vi "Timer Core.vi"(0 "timer":T2, 1 "function":T3(ring)=enum."test ref", 5 "return exisiting (F)":bool, 7 "Accuracy":enum16{"1 ms", "10 ms"}(ring), 9 "name":string, 11 "error in (no error)":errorcluster, 12 "Wait timeout [sec]":dbl format="%.3f") -> (2 "error":i32, 4 "timer out":T2, 6 "Keep Waiting":bool, 8 "Timers out":T1(array[cluster]) {"Total time [sec]" format="%.3f"; "Start time [sec]" format="%.3f"}, 10 "name out":string, 14 "message out":string, 15 "error out":errorcluster)   [LabVIEW 2011]
uses:
  Timer Refnum.ctl
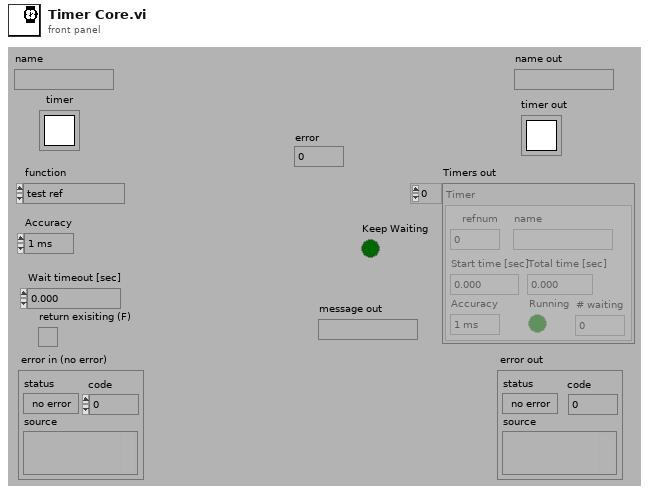
[diagram p1: front panel]
types:
  T1 = cluster{"refnum":u32, "Start time [sec]":dbl, "Running":bool, "Total time [sec]":dbl, "name":string, "Accuracy":enum16{"1 ms", "10 ms"}, "# waiting":i32}[]
  T2 = typedef "Timer Refnum.ctl" = refnum<k1>
  T3 = enum16{"open ref", "lookup ref", "close ref", "test ref", "start", "stop", "wait", "reset", "increment # waiting", "decrement #waiting"}
  T4 = enum16{"open ref", "lookup ref", "close ref", "test ref", "start", "stop", "wait", "reset"}
  T5 = cluster{"refnum":u32, "Start time (s)":dbl, "Running":bool, "Total time (s)":dbl, "name":string, "Accuracy":enum16{"1 ms", "10 ms"}, "# waiting":i32}
  T6 = cluster{"refnum":u32, "Start time (s)":dbl, "Running":bool, "Total time (s)":dbl, "name":string, "Accuracy":enum16{"1 ms", "10 ms"}, "# waiting":i32}[]
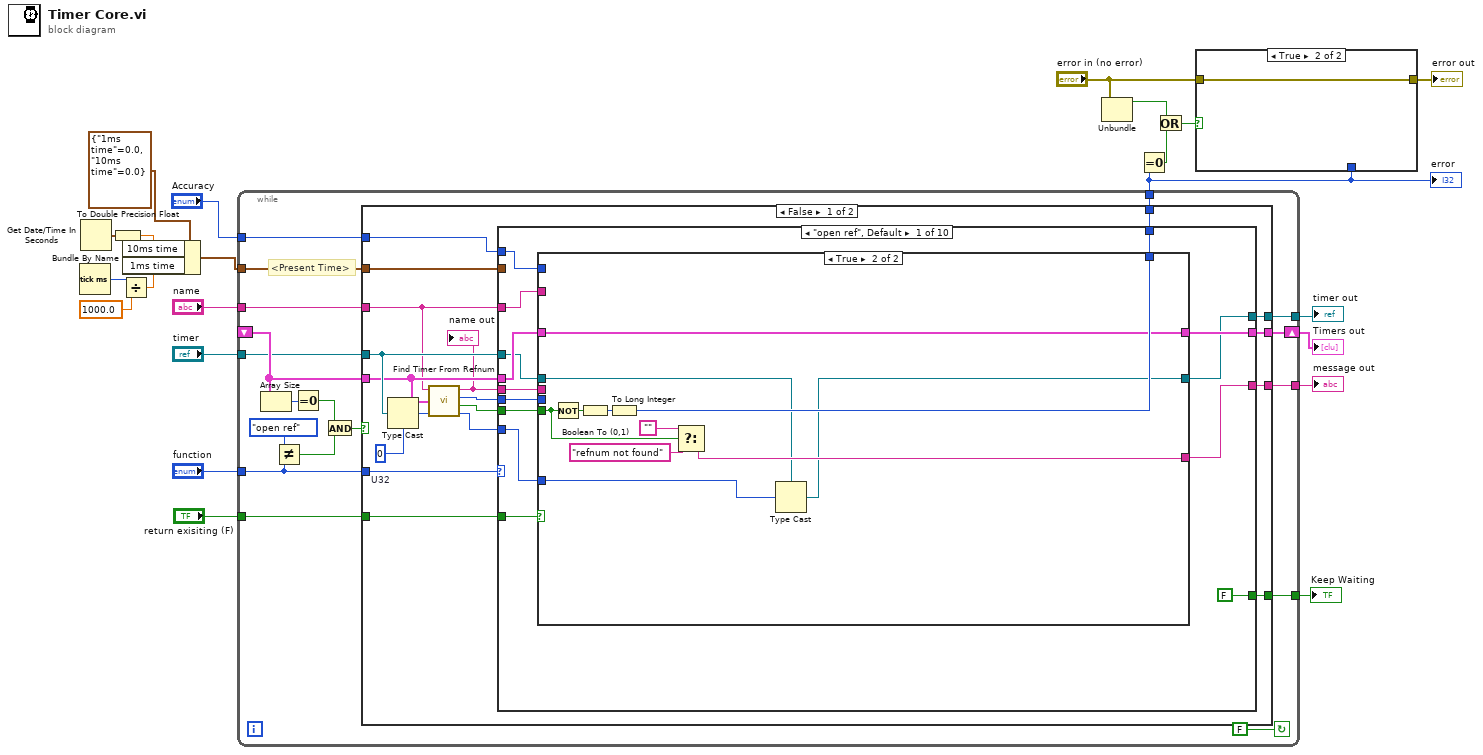
[diagram p0: block diagram]
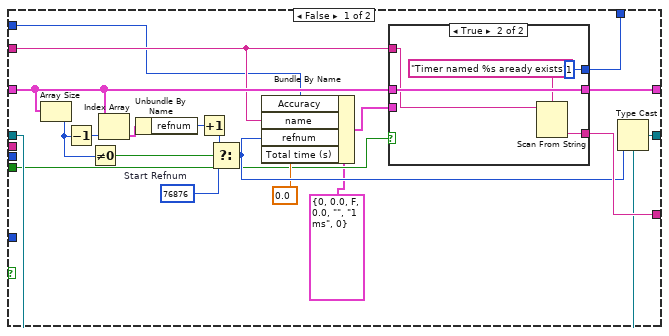
[diagram p2: hidden frame]
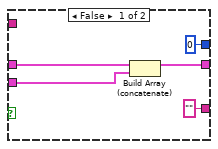
[diagram p3: hidden frame]
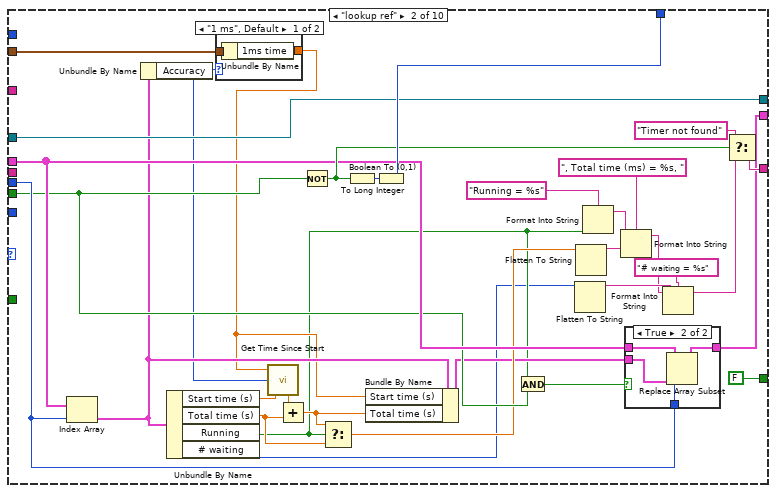
[diagram p4: hidden frame]
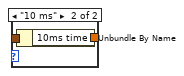
[diagram p5: hidden frame]
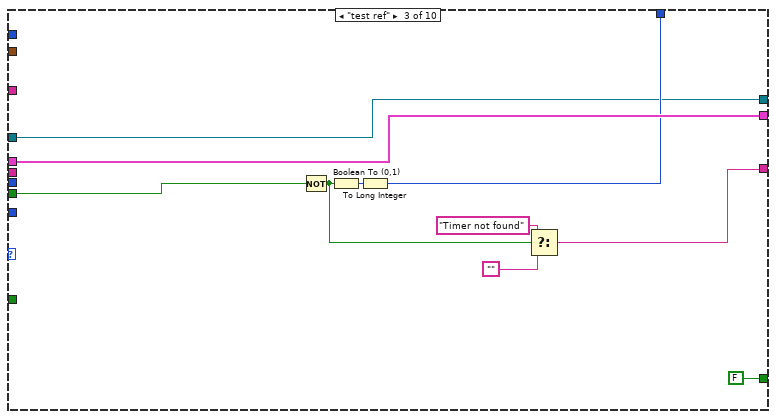
[diagram p7: hidden frame]
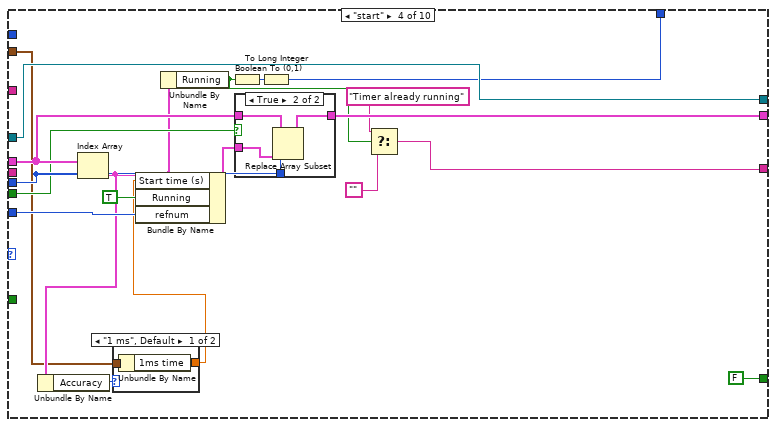
[diagram p8: hidden frame]
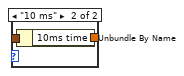
[diagram p9: hidden frame]
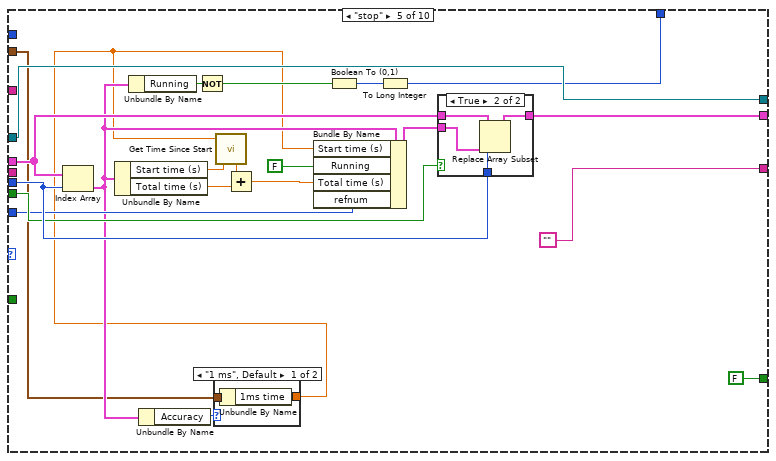
[diagram p11: hidden frame]
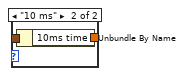
[diagram p12: hidden frame]
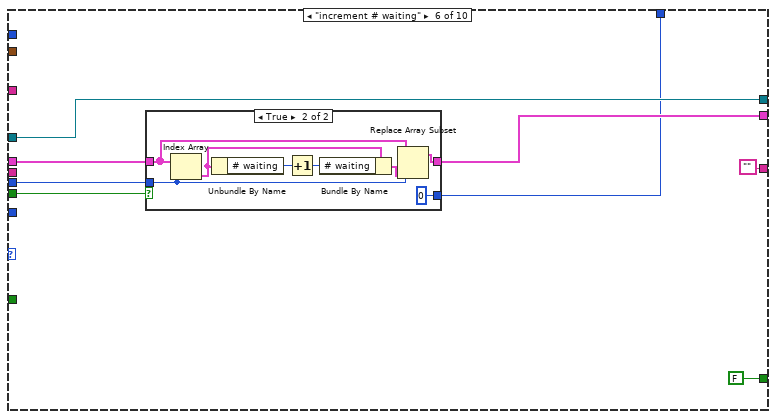
[diagram p14: hidden frame]
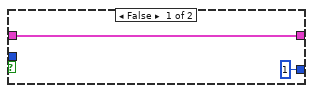
[diagram p15: hidden frame]
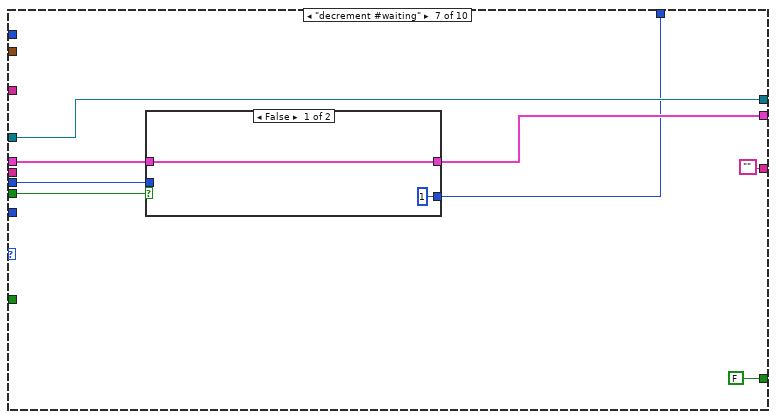
[diagram p16: hidden frame]
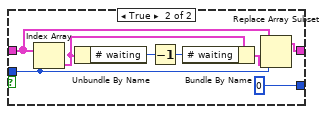
[diagram p17: hidden frame]
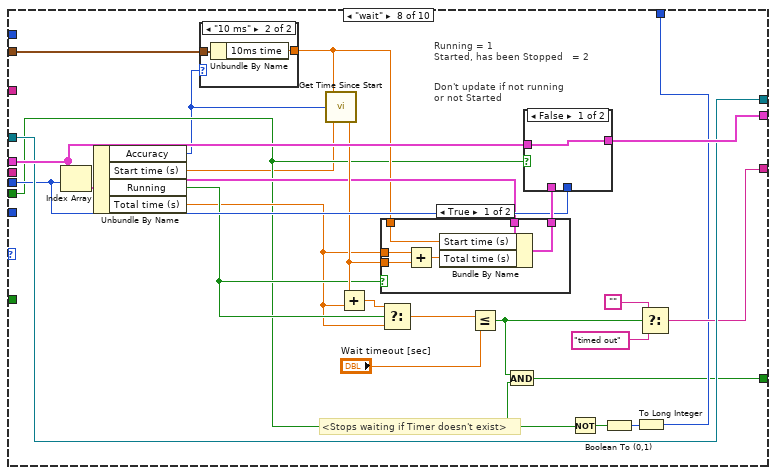
[diagram p18: hidden frame]
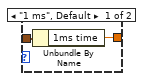
[diagram p19: hidden frame]
diagram:
  n1 = Tick Count (ms)() -> (millisecond timer value=w6:u32)
  n2 = Get Date/Time In Seconds() -> (seconds since 1Jan1904=w1:timestamp)
  n3 = To Double Precision Float(number=w1) -> (double precision float=w8:dbl)
  n4 = Divide(x=w6, y=1000.0) -> (x/y=w4:dbl)
  n5 = Bundle By Name(cluster=cluster{"1ms time":dbl, "10ms time":dbl} {"1ms time"=0.0, "10ms time"=0.0} ("Source Element"), "10ms time"=w8, "1ms time"=w4) -> (w7:cluster{"1ms time":dbl, "10ms time":dbl})
  n6 = while {
    tunnel: "Accuracy" -> [w24]
    tunnel: [w25] -> w9
    tunnel: "function" -> [w26]
    tunnel: "return exisiting (F)" -> [w27]
    tunnel: w7 -> [w30]
    tunnel: [w32] -> w13
    tunnel: [w33] -> w15
    tunnel: "name" -> [w34]
    tunnel: [w35] -> w10
    tunnel: "timer" -> [w29]
    shift-left: _ -> [w40]
    shift-right: [w28] -> w14
    stop <- FALSE continue-if-true
    # "<Present Time>"
    n7 = Array Size(array=w40) -> (size(s)=w39:i32)
    n8 = Not Equal?(x=T4."open ref" ("function"), y=w26) -> (x != y?=w37:bool)
    n9 = Equal To 0?(x=w39) -> (x = 0?=w36:bool)
    n10 = And(x=w36, y=w37) -> (x .and. y?=w38:bool)
    n11 = case shown="False" w38 {
      tunnel: w40 -> [w49 w333]
      tunnel: w26 -> [w58 _]
      tunnel: [w57 1 ("index")] -> w35
      tunnel: w34 -> [w43 _]
      tunnel: [w56 ""] -> w33
      tunnel: [w55 w335] -> w32
      tunnel: w30 -> [w54 _]
      tunnel: w29 -> [w50 w335]
      tunnel: [w53 w333] -> w28
      tunnel: w27 -> [w52 _]
      tunnel: [w42 FALSE ("f")] -> w25
      tunnel: w24 -> [w41 _]
      frame False {
        w51 = u32 0  # U32
        n12 = Type Cast(type=w51, x=w50) -> (*(type *) &x=w44:u32)
        n13 = call "Find Timer From Refnum.vi"("Timers out"=w49, "timer refnum"=w44, "timer name"=w43) -> ("timer refnum out"=w45:u32, "Found"=w48:bool, "timer index"=w47:i32, "name out"=w46:string)  [unwired: 2 in]
        "name out" <- w46
        n14 = case shown="\"open ref\", Default" w58 {
          tunnel: w49 -> [w72 w131 w164 w178 w203 w226 w244 w283 w306 w323]
          tunnel: [w71 w132 w164 w182 w212 w225 w243 w282 w311 w324] -> w53
          tunnel: w50 -> [w65 w143 w161 w181 w211 w231 w249 w281 w310 w331]
          tunnel: [w70 w144 w162 w179 w204 w224 w242 w275 w308 0 ("x")] -> w57
          tunnel: w43 -> [w68 _ _ _ _ _ _ _ _ _]
          tunnel: [w69 w138 w158 w170 "" "" "" w278 "" ""] -> w56
          tunnel: [w67 w143 w161 w181 w211 w231 w249 w281 w310 w331] -> w55
          tunnel: w54 -> [_ w127 _ w165 w194 _ _ w267 _ _]
          tunnel: w52 -> [w66 _ _ _ _ _ _ _ _ _]
          tunnel: w46 -> [w62 _ _ _ _ _ _ _ _ _]
          tunnel: w48 -> [w64 w130 w159 w176 w201 w228 w246 w264 w303 _]
          tunnel: w45 -> [w59 _ _ w175 w198 _ _ _ w305 _]
          tunnel: w47 -> [w63 w133 _ w177 w202 w227 w245 w274 w304 w321]
          tunnel: [FALSE ("f") FALSE ("f") FALSE ("f") FALSE ("f") FALSE ("f") FALSE ("f") FALSE ("f") w262 FALSE ("f") FALSE ("f")] -> w42
          tunnel: w41 -> [w60 _ _ _ _ _ _ _ _ _]
          frame "open ref", Default {
            n15 = case shown="True" w66 {
              tunnel: w72 -> [w92 w106]
              tunnel: [w83 w106] -> w71
              tunnel: [w82 w112] -> w70
              tunnel: [w81 w107] -> w69
              tunnel: w68 -> [w80 _]
              tunnel: [w78 w103] -> w67
              tunnel: w65 -> [w77 w104]
              tunnel: w64 -> [w75 w110]
              tunnel: w63 -> [_ _]
              tunnel: w62 -> [_ _]
              tunnel: w60 -> [w73 _]
              tunnel: w59 -> [_ w105]
              frame False {
                w85 = u32 76876  # Start Refnum
                n16 = Array Size(array=w92) -> (size(s)=w88:i32)
                n17 = Decrement(x=w88) -> (x-1=w91:i32)
                n18 = Not Equal To 0?(x=w88) -> (x != 0?=w87:bool)
                n19 = Index Array(array=w92, index=w91) -> (element=w90:T5)
                n20 = Unbundle By Name(w90) -> ("refnum"=w89:u32)
                n21 = Increment(x=w89) -> (x+1=w86:u32)
                n22 = Select(t=w86, s=w87, f=w85) -> (s? t:f=w79:u32)
                n23 = Bundle By Name(cluster=T5 {"refnum"=0, "Start time (s)"=0.0, "Running"=FALSE, "Total time (s)"=0.0, "name"="", "Accuracy"=enum."1 ms", "# waiting"=0} ("Timer"), "Accuracy"=w73, "name"=w80, "refnum"=w79, "Total time (s)"=0.0 ("Bundle Element")) -> (w84:T5)
                n24 = case shown="True" w75 {
                  tunnel: w92 -> [w97 w102]
                  tunnel: w84 -> [w96 _]
                  tunnel: [w95 w102] -> w83
                  tunnel: [0 ("x") 1 ("x")] -> w82
                  tunnel: ["" w100] -> w81
                  tunnel: w80 -> [_ w99]
                  frame False {
                    n25 = Build Array (concatenate)(w97, w96) -> (w95:T6)
                  }
                  frame True {
                    n26 = Scan From String(format string="Timer named %s aready exists" ("Format String"), input string=w99) -> (output 1=w100:string)  [unwired: 3 in, 3 out]
                  }
                }
                n27 = Type Cast(type=w77, x=w79) -> (*(type *) &x=w78:T2)
              }
              frame True {
                n28 = Not(x=w110) -> (.not. x?=w111:bool)
                n29 = Boolean To (0,1)(Boolean=w111) -> (0, 1=w113:i16)
                n30 = To Long Integer(number=w113) -> (32bit integer=w112:i32)
                n31 = Select(t="", s=w110, f="refnum not found") -> (s? t:f=w107:string)
                n32 = Type Cast(type=w104, x=w105) -> (*(type *) &x=w103:T2)
              }
            }
          }
          frame "lookup ref" {
            n33 = Index Array(array=w131, index=w133) -> (element=w126:T5)
            n34 = Unbundle By Name(w126) -> ("Accuracy"=w124:enum16{"1 ms", "10 ms"})
            n35 = Unbundle By Name(w126) -> ("Start time (s)"=w134:dbl, "Total time (s)"=w123:dbl, "Running"=w119:bool, "# waiting"=w118:i32)
            n36 = case shown="\"1 ms\", Default" w124 {
              tunnel: w127 -> [w147 w149]
              tunnel: [w146 w148] -> w125
              frame "1 ms", Default {
                n37 = Unbundle By Name(w147) -> ("1ms time"=w146:dbl)
              }
              frame "10 ms" {
                n38 = Unbundle By Name(w149) -> ("10ms time"=w148:dbl)
              }
            }
            n39 = call "Get Time Since Start.vi"("Start time (s)"=w134, "Accuracy"=w124, "Time now (s)"=w125) -> ("Difference"=w135:dbl)
            n40 = Add(x=w135, y=w123) -> (x+y=w122:dbl)
            n41 = Not(x=w130) -> (.not. x?=w137:bool)
            n42 = Select(t=w122, s=w119, f=w123) -> (s? t:f=w121:dbl)
            n43 = Boolean To (0,1)(Boolean=w137) -> (0, 1=w145:i16)
            n44 = Bundle By Name(cluster=w126, "Start time (s)"=w125, "Total time (s)"=w122) -> (w120:T5)
            n45 = To Long Integer(number=w145) -> (32bit integer=w144:i32)
            n46 = And(x=w119, y=w130) -> (x .and. y?=w129:bool)
            n47 = Flatten To String(anything=w118) -> (data string=w117:string)  [unwired: 3 in, 2 out]
            n48 = Flatten To String(anything=w121) -> (data string=w139:string)  [unwired: 3 in, 2 out]
            n49 = Format Into String(format string="Running = %s" ("Format String"), w119) -> (resulting string=w141:string)  [unwired: 2 in, 1 out]
            n50 = Format Into String(format string=", Total time (ms) = %s, " ("Format String"), initial string=w141, w139) -> (resulting string=w116:string)  [unwired: 1 in, 1 out]
            n51 = case shown="True" w129 {
              tunnel: w120 -> [_ w154]
              tunnel: [w150 w153] -> w132
              tunnel: w131 -> [w150 w152]
              tunnel: w133 -> [_ w151]
              frame False {
              }
              frame True {
                n52 = Replace Array Subset(array=w152, new element=w154, index=w151) -> (w153:T6)
              }
            }
            n53 = Format Into String(format string="# waiting = %s" ("Format String"), initial string=w116, w117) -> (resulting string=w114:string)  [unwired: 1 in, 1 out]
            n54 = Select(t="Timer not found" ("f"), s=w137, f=w114) -> (s? t:f=w138:string)
          }
          frame "test ref" {
            n55 = Not(x=w159) -> (.not. x?=w156:bool)
            n56 = Boolean To (0,1)(Boolean=w156) -> (0, 1=w163:i16)
            n57 = To Long Integer(number=w163) -> (32bit integer=w162:i32)
            n58 = Select(t="Timer not found" ("f"), s=w156, f="") -> (s? t:f=w158:string)
          }
          frame "start" {
            n59 = Index Array(array=w178, index=w177) -> (element=w166:T5)
            n60 = Unbundle By Name(w166) -> ("Accuracy"=w168:enum16{"1 ms", "10 ms"})
            n61 = case shown="\"1 ms\", Default" w168 {
              tunnel: w165 -> [w185 w187]
              tunnel: [w184 w186] -> w167
              frame "1 ms", Default {
                n62 = Unbundle By Name(w185) -> ("1ms time"=w184:dbl)
              }
              frame "10 ms" {
                n63 = Unbundle By Name(w187) -> ("10ms time"=w186:dbl)
              }
            }
            n64 = Bundle By Name(cluster=w166, "Start time (s)"=w167, "Running"=TRUE ("Bundle Element"), "refnum"=w175) -> (w183:T5)
            n65 = Unbundle By Name(w166) -> ("Running"=w173:bool)
            n66 = Boolean To (0,1)(Boolean=w173) -> (0, 1=w180:i16)
            n67 = case shown="True" w176 {
              tunnel: w183 -> [_ w192]
              tunnel: w177 -> [_ w191]
              tunnel: w178 -> [w188 w190]
              tunnel: [w188 w189] -> w182
              frame False {
              }
              frame True {
                n68 = Replace Array Subset(array=w190, new element=w192, index=w191) -> (w189:T6)
              }
            }
            n69 = To Long Integer(number=w180) -> (32bit integer=w179:i32)
            n70 = Select(t="Timer already running", s=w173, f="") -> (s? t:f=w170:string)
          }
          frame "stop" {
            n71 = Index Array(array=w203, index=w202) -> (element=w195:T5)
            n72 = Unbundle By Name(w195) -> ("Start time (s)"=w199:dbl, "Total time (s)"=w209:dbl)
            n73 = Unbundle By Name(w195) -> ("Running"=w207:bool)
            n74 = Unbundle By Name(w195) -> ("Accuracy"=w196:enum16{"1 ms", "10 ms"})
            n75 = Not(x=w207) -> (.not. x?=w205:bool)
            n76 = case shown="\"1 ms\", Default" w196 {
              tunnel: w194 -> [w216 w218]
              tunnel: [w215 w217] -> w193
              frame "1 ms", Default {
                n77 = Unbundle By Name(w216) -> ("1ms time"=w215:dbl)
              }
              frame "10 ms" {
                n78 = Unbundle By Name(w218) -> ("10ms time"=w217:dbl)
              }
            }
            n79 = call "Get Time Since Start.vi"("Start time (s)"=w199, "Time now (s)"=w193) -> ("Difference"=w200:dbl)  [unwired: 1 in]
            n80 = Add(x=w200, y=w209) -> (x+y=w208:dbl)
            n81 = Bundle By Name(cluster=w195, "Start time (s)"=w193, "Running"=FALSE ("Bundle Element"), "Total time (s)"=w208, "refnum"=w198) -> (w213:T5)
            n82 = Boolean To (0,1)(Boolean=w205) -> (0, 1=w206:i16)
            n83 = To Long Integer(number=w206) -> (32bit integer=w204:i32)
            n84 = case shown="True" w201 {
              tunnel: w213 -> [_ w223]
              tunnel: [w219 w222] -> w212
              tunnel: w203 -> [w219 w221]
              tunnel: w202 -> [_ w220]
              frame False {
              }
              frame True {
                n85 = Replace Array Subset(array=w221, new element=w223, index=w220) -> (w222:T6)
              }
            }
          }
          frame "increment # waiting" {
            n86 = case shown="True" w228 {
              tunnel: w226 -> [w233 w238]
              tunnel: w227 -> [_ w236]
              tunnel: [w233 w235] -> w225
              tunnel: [1 ("timer index") 0 ("timer index")] -> w224
              frame False {
              }
              frame True {
                n87 = Index Array(array=w238, index=w236) -> (element=w240:T5)
                n88 = Unbundle By Name(w240) -> ("# waiting"=w241:i32)
                n89 = Increment(x=w241) -> (x+1=w239:i32)
                n90 = Bundle By Name(cluster=w240, "# waiting"=w239) -> (w237:T5)
                n91 = Replace Array Subset(array=w238, new element=w237, index=w236) -> (w235:T6)
              }
            }
          }
          frame "decrement #waiting" {
            n92 = case shown="False" w246 {
              tunnel: w244 -> [w251 w256]
              tunnel: w245 -> [_ w254]
              tunnel: [w251 w253] -> w243
              tunnel: [1 ("timer index") 0 ("timer index")] -> w242
              frame False {
              }
              frame True {
                n93 = Index Array(array=w256, index=w254) -> (element=w258:T5)
                n94 = Unbundle By Name(w258) -> ("# waiting"=w259:i32)
                n95 = Decrement(x=w259) -> (x-1=w257:i32)
                n96 = Bundle By Name(cluster=w258, "# waiting"=w257) -> (w255:T5)
                n97 = Replace Array Subset(array=w256, new element=w255, index=w254) -> (w253:T6)
              }
            }
          }
          frame "wait" {
            # "Running = 1\nStarted, has been Stopped   = 2"
            # "Don't update if not running\nor not Started"
            # "<Stops waiting if Timer doesn't exist>"
            n98 = Index Array(array=w283, index=w274) -> (element=w268:T5)
            n99 = Unbundle By Name(w268) -> ("Accuracy"=w260:enum16{"1 ms", "10 ms"}, "Start time (s)"=w261:dbl, "Running"=w270:bool, "Total time (s)"=w269:dbl)
            n100 = case shown="\"10 ms\"" w260 {
              tunnel: w267 -> [w286 w288]
              tunnel: [w285 w287] -> w266
              frame "1 ms", Default {
                n101 = Unbundle By Name(w286) -> ("1ms time"=w285:dbl)
              }
              frame "10 ms" {
                n102 = Unbundle By Name(w288) -> ("10ms time"=w287:dbl)
              }
            }
            n103 = call "Get Time Since Start.vi"("Start time (s)"=w261, "Accuracy"=w260, "Time now (s)"=w266) -> ("Difference"=w273:dbl)
            n104 = Add(x=w273, y=w269) -> (x+y=w272:dbl)
            n105 = case shown="True" w270 {
              tunnel: [w294 w295] -> w284
              tunnel: w268 -> [w293 w295]
              tunnel: w269 -> [w292 _]
              tunnel: w273 -> [w291 _]
              tunnel: w266 -> [w289 _]
              frame True {
                n106 = Add(x=w292, y=w291) -> (x+y=w290:dbl)
                n107 = Bundle By Name(cluster=w293, "Start time (s)"=w289, "Total time (s)"=w290) -> (w294:T5)
              }
              frame False {
              }
            }
            n108 = Select(t=w272, s=w270, f=w269) -> (s? t:f=w271:dbl)
            n109 = Less Or Equal?(x=w271, y="Wait timeout [sec]") -> (x <= y?=w263:bool)
            n110 = And(x=w263, y=w264) -> (x .and. y?=w262:bool)
            n111 = case shown="False" w264 {
              tunnel: w284 -> [_ w300]
              tunnel: w274 -> [_ w299]
              tunnel: w283 -> [w296 w298]
              tunnel: [w296 w297] -> w282
              frame False {
              }
              frame True {
                n112 = Replace Array Subset(array=w298, new element=w300, index=w299) -> (w297:T6)
              }
            }
            n113 = Not(x=w264) -> (.not. x?=w277:bool)
            n114 = Boolean To (0,1)(Boolean=w277) -> (0, 1=w276:i16)
            n115 = To Long Integer(number=w276) -> (32bit integer=w275:i32)
            n116 = Select(t="", s=w263, f="timed out") -> (s? t:f=w278:string)
          }
          frame "reset" {
            w302 = 0.0 ("Bundle Element")
            n117 = Index Array(array=w306, index=w304) -> (element=w307:T5)
            n118 = Bundle By Name(cluster=w307, "refnum"=w305, "Start time (s)"=w302, "Running"=FALSE ("Bundle Element"), "Total time (s)"=w302) -> (w312:T5)
            n119 = case shown="True" w303 {
              tunnel: w312 -> [_ w320]
              tunnel: [w315 w319] -> w311
              tunnel: w306 -> [w315 w318]
              tunnel: w304 -> [_ w317]
              tunnel: [1 ("x") 0 ("x")] -> w308
              frame False {
              }
              frame True {
                n120 = Replace Array Subset(array=w318, new element=w320, index=w317) -> (w319:T6)
              }
            }
          }
          frame "close ref" {
            n121 = Split 1D Array(array=w323, index=w321) -> (first subarray=w325:T6, second subarray=w328:T6)
            n122 = Split 1D Array(array=w328, index=1) -> (second subarray=w326:T6)  [unwired: 1 out]
            n123 = Build Array (concatenate)(w325, w326) -> (w324:T6)
          }
        }
      }
      frame True {
      }
    }
  }
  "timer out" <- w13
  "error" <- w10
  "message out" <- w15
  "Timers out" <- w14
  "Keep Waiting" <- w9
  n124 = Unbundle("error in (no error)") -> ("status"=w20:bool)  [unwired: 2 out]
  n125 = Equal To 0?(x=w10) -> (x = 0?=w19:bool)
  n126 = Or(x=w20, y=w19) -> (x .or. y?=w18:bool)
  n127 = case shown="True" w18 {
    tunnel: "error in (no error)" -> [w345 w348]
    tunnel: [w344 w348] -> w22
    tunnel: w10 -> [w342 _]
    frame False {
      n128 = Call Chain() -> (call chain=w340:string[])
      n129 = Split 1D Array(array=w340, index=1) -> (second subarray=w338:string[])  [unwired: 1 out]
      n130 = Reverse 1D Array(array=w338) -> (reversed array=w337:string[])
      n131 = Array To Spreadsheet String(delimiter (Tab)=" >> ", array=w337, 3:"%s" ("format string")) -> (spreadsheet string=w343:string)
      n132 = Bundle(cluster=w345, "status"=TRUE, "code"=w342, "source"=w343) -> (w344:errorcluster)
    }
    frame True {
    }
  }
  "error out" <- w22
